vi "Omron_FCS.vi"(1 "Command":string) -> (0 "FCS":string)   [LabVIEW 2015]
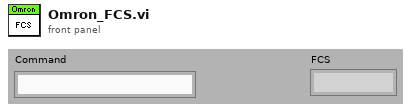
[diagram p1: front panel]
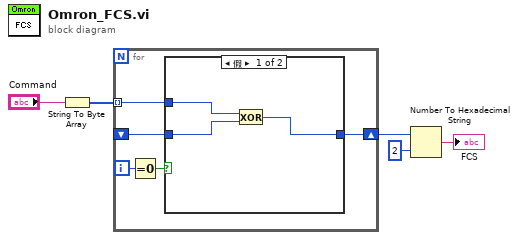
[diagram p0: block diagram]
diagram:
  n1 = String To Byte Array(string="Command") -> (unsigned byte array=w5:u8[])
  n2 = for {
    tunnel: w5 -> [w9] mode=indexing
    shift-right: [w7] -> w4
    shift-left: _ -> [w6]
    i -> [w10]
    n3 = Equal To 0?(x=w10) -> (x = 0?=w8:bool)
    n4 = case shown="假" w8 {
      tunnel: w9 -> [w13 w14]
      tunnel: [w11 w14] -> w7
      tunnel: w6 -> [w12 _]
      frame False {
        n5 = Exclusive Or(1:w12, 2:w13) -> (0:w11:u8)
      }
      frame True {
      }
    }
  }
  n6 = Number To Hexadecimal String(1:i16 2 ("width (-)"), 2:w4) -> (0:→"FCS":string)
